vi "Add TX Count.vi"(8 "error in (no error)":errorcluster, 9 "Add (1)":i32=1, 10 "Connection Name":string, 11 "VectoService in":refnum<class "VectoInfo.lvclass">) -> (0 "error out":errorcluster, 3 "VectoService out":refnum<class "VectoInfo.lvclass">)   [LabVIEW 2020, in "Vecto.lvlib" / "VectoInfo.lvclass"]
uses:
  VectoInfo.lvclass
  Count Data.ctl
  VectoInfo.lvclass/VectoInfo.ctl
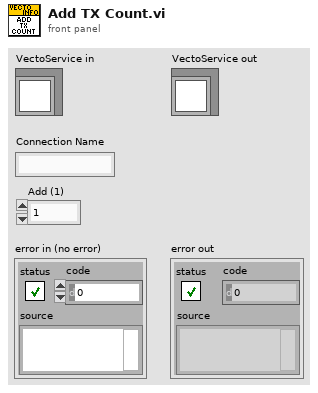
[diagram p1: front panel]
types:
  T1 = typedef "Vecto.lvlib/VectoInfo.lvclass/Count Data.ctl" = cluster{"Name":string, "Amount":i32}
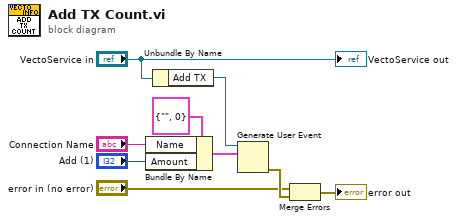
[diagram p0: block diagram]
diagram:
  n1 = Bundle By Name(cluster=T1 {"Name"="", "Amount"=0} ("Count Data"), "Name"="Connection Name", "Amount"="Add (1)") -> (w6:T1)
  n2 = Unbundle By Name("VectoService in") -> ("Add TX"=w5:refnum<user-event>)
  n3 = Generate User Event(user event=w5, event data cluster=w6) -> (error out=w4:errorcluster)  [unwired: 2 in, 1 out]
  n4 = Merge Errors("error in (no error)", w4) -> (→"error out":errorcluster)
  "VectoService out" <- "VectoService in"
